vi "Get Outputs Definition.vi"(11 "Outputs":refnum<class "Terminal.lvclass">[](array[class])) -> (2 "Default Output":variant, 3 "output string":string)   [LabVIEW 2019, in "Terminal.lvclass"]
doc: "JKI State Machine Objects (SMO) 1.3.0.56\nJKI - JKI\nCopyright (c) 2017, JKI"
uses:
  Terminal.lvclass
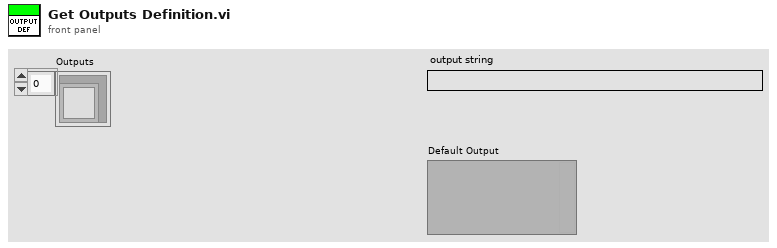
[diagram p1: front panel]
types:
  T1 = typedef "VariantType.lvlib/Type.ctl" = enum8{"Invalid Type", "Void", "I8", "I16", "I32", "I64", "U8", "U16", "U32", "U64", "Single Float", "Double Float", "Extended Float", "Single Complex", "Double Complex", "Extended Complex", "Enum U8", "Enum U16", "Enum U32", "Enum U64", "Single Float With Unit", "Double Float With Unit", "Extended Float With Unit", "Single Complex with Unit", "Double Complex with Unit", "Extended Complex with Unit", "Boolean", "String", "Path", "Picture", "Tag", "Array", "Cluster", "Variant", "LV Variant", "Waveform", "Timestamp", "Digital Waveform", "Digital Data", "ExpressData", "Refnum", "External Data", "VI", "Poly VI", "LabVIEW Class Instance", "Fixed Point"}
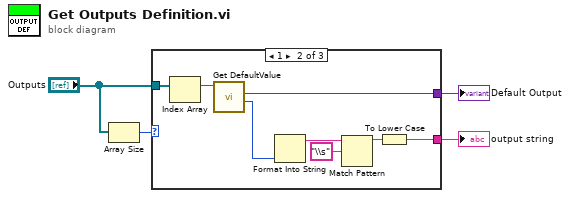
[diagram p0: block diagram]
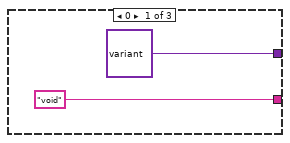
[diagram p2: hidden frame]
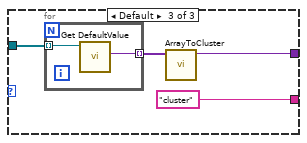
[diagram p3: hidden frame]
diagram:
  n1 = Array Size(array="Outputs") -> (size(s)=w4:i32)
  n2 = case shown="1" w4 {
    tunnel: "Outputs" -> [_ w14 w17]
    tunnel: ["void" w13 "cluster"] -> w2
    tunnel: [variant ("Default Value") w8 w15] -> w1
    frame 0 {
    }
    frame 1 {
      n3 = Index Array(array=w14) -> (element=w9:refnum<class "Terminal.lvclass">)  [unwired: 1 in]
      n4 = call "Get DefaultValue.vi"("Terminal in"=w9) -> ("Type Enum"=w7:T1, "Default Value"=w8:variant)  [unwired: 7 in, 2 out]
      n5 = Format Into String(w7) -> (resulting string=w11:string)  [unwired: 3 in, 1 out]
      n6 = Match Pattern(string=w11, regular expression="\\s") -> (before substring=w10:string)  [unwired: 1 in, 3 out]
      n7 = To Lower Case(string=w10) -> (all lower case string=w13:string)
    }
    frame Default {
      n8 = for {
        tunnel: w17 -> [w20] mode=indexing
        tunnel: [w19] -> w16 mode=indexing
        n9 = call "Get DefaultValue.vi"("Terminal in"=w20) -> ("Default Value"=w19:variant)  [unwired: 7 in, 3 out]
      }
      n10 = call "ArrayToCluster.vi"("Array"=w16) -> ("Cluster"=w15:variant)  [unwired: 10 in]
    }
  }
  "Default Output" <- w1
  "output string" <- w2
